vi "Acquire.vi"(6 "Infm Alive Counter":u16, 7 "Signal Type":T4, 8 "error in (no error)":errorcluster, 9 "WiBCI16T Data":T1 {"Reg Map"."ADS2" format="%x"; "Reg Map"."ADS1" format="%x"}, 11 "connection UDP":refnum<k16>) -> (0 "error out":errorcluster, 1 "Data Valid ?":bool, 2 "WiBCI16T Data out":T1 {"Reg Map"."ADS2" format="%x"; "Reg Map"."ADS1" format="%x"}, 3 "connection ID out":refnum<k16>, 4 "Infm Alive Counter out":u16)   [LabVIEW 2019, in "Acquisition.lvlib"]
doc: "Perform the acquisition. Replace the contents of this diagram with calls to acquisition hardware.\n_____\nBased on DQMH Project Template 6.1.0.94."
uses:
  Acquisition.lvlib
  Signal Type--enum.ctl
  WiBCI16T_Data.ctl
  WiBCI16T_Status.ctl
  Reg_Map.ctl
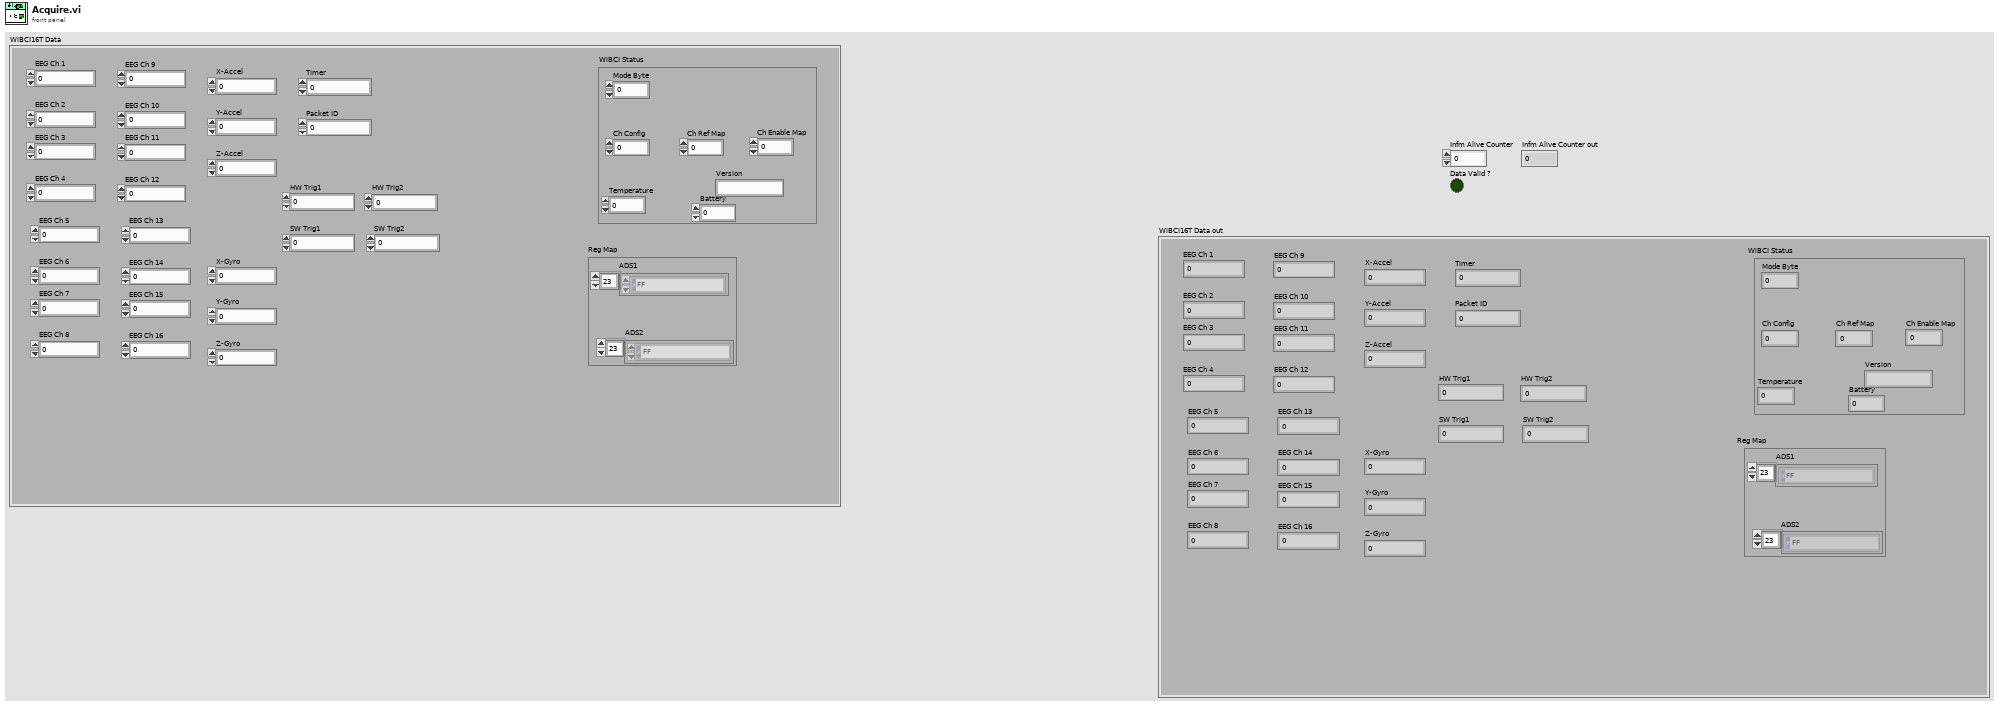
[diagram p1: front panel]
types:
  T1 = typedef "Acquisition.lvlib/WiBCI16T_Data.ctl" = cluster{"EEG Ch 1":dbl, "EEG Ch 2":dbl, "EEG Ch 3":dbl, "EEG Ch 4":dbl, "EEG Ch 5":dbl, "EEG Ch 6":dbl, "EEG Ch 7":dbl, "EEG Ch 8":dbl, "EEG Ch 9":dbl, "EEG Ch 10":dbl, "EEG Ch 11":dbl, "EEG Ch 12":dbl, "EEG Ch 13":dbl, "EEG Ch 14":dbl, "EEG Ch 15":dbl, "EEG Ch 16":dbl, "X-Accel":i16, "Y-Accel":i16, "Z-Accel":i16, "X-Gyro":i16, "Y-Gyro":i16, "Z-Gyro":i16, "Timer":u32, "Packet ID":u32, "HW Trig1":u8, "SW Trig1":i8, "HW Trig2":u8, "SW Trig2":i8, "WiBCI Status":T2, "Reg Map":T3}
  T2 = typedef "Acquisition.lvlib/WiBCI16T_Status.ctl" = cluster{"Mode Byte":u8, "Ch Config":u8, "Ch Ref Map":u16, "Ch Enable Map":u16, "Temperature":sgl, "Battery":u8, "Version":string}
  T3 = typedef "Acquisition.lvlib/Reg_Map.ctl" = cluster{"ADS1":u8[], "ADS2":u8[]}
  T4 = typedef "Acquisition.lvlib/Signal Type--enum.ctl" = enum16{"Sine Wave", "Square with Noise"}
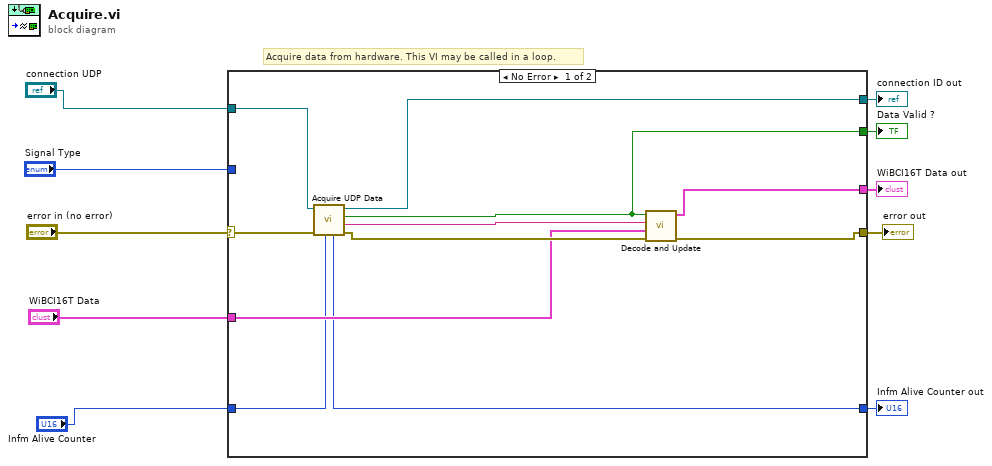
[diagram p0: block diagram]
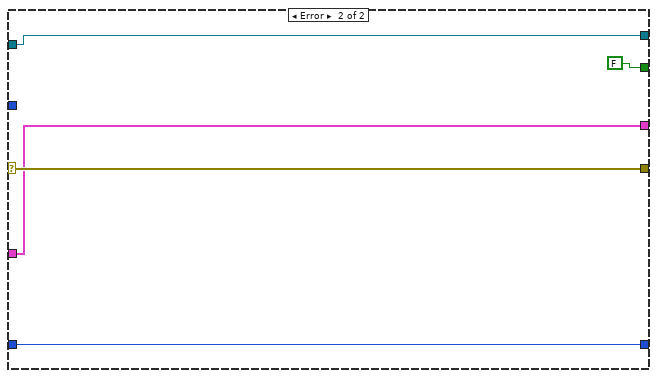
[diagram p2: hidden frame]
diagram:
  # "Acquire data from hardware. This VI may be called in a loop."
  n1 = case shown="No Error" "error in (no error)" {
    selector: "error in (no error)" -> [w21 w26]
    tunnel: [w17 w26] -> w9
    tunnel: "Signal Type" -> [_ _]
    tunnel: "connection UDP" -> [w20 w25]
    tunnel: [w19 w25] -> w6
    tunnel: "WiBCI16T Data" -> [w15 w24]
    tunnel: [w14 w24] -> w4
    tunnel: "Infm Alive Counter" -> [w12 w22]
    tunnel: [w13 FALSE] -> w2
    tunnel: [w11 w22] -> w1
    frame No Error {
      n2 = call "Acquire UDP Data.vi"("Infm Alive Counter"=w12, "error in"=w21, "connection UDP in"=w20) -> ("error out"=w18:errorcluster, "data out"=w16:string, "Data Valid ?"=w13:bool, "connection ID out"=w19:refnum<k16>, "Infm Alive Counter out"=w11:u16)  [unwired: 4 in]
      n3 = call "Decode and Update.vi"("error in"=w18, "WiBCI16T Data"=w15, "data in"=w16, "Data Valid ?"=w13) -> ("error out"=w17:errorcluster, "WiBCI16T Data out"=w14:T1)  [unwired: 6 in]
    }
    frame Error {
    }
  }
  "error out" <- w9
  "connection ID out" <- w6
  "WiBCI16T Data out" <- w4
  "Data Valid ?" <- w2
  "Infm Alive Counter out" <- w1
